vi "closeConfigFile.vi"(8 "error in (no error)":errorcluster, 11 "Path in":T1) -> (0 "error out":errorcluster)   [LabVIEW 2018]
doc: "Close the default.ini file.\n\nNOTE: this is only for internal use. User does not call this function directly."
uses:
  <vilib>/Utility/config.llb/Config Data RefNum.ctl
  <vilib>/Utility/config.llb/NI_LVConfig.lvlib
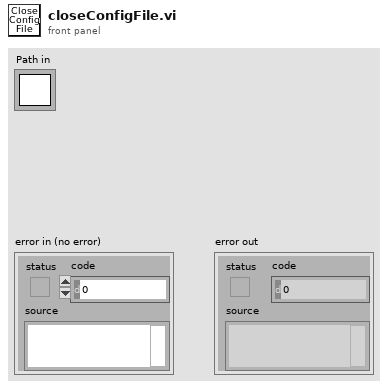
[diagram p1: front panel]
types:
  T1 = typedef "NI_LVConfig.lvlib/Config Data RefNum.ctl" = refnum<k1>
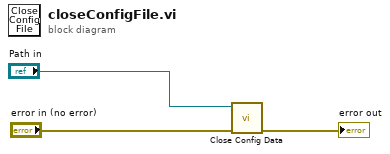
[diagram p0: block diagram]
diagram:
  n1 = call <vilib>:"Close Config Data.vi"("error in (no error)"="error in (no error)", "refnum"="Path in") -> ("error out"=→"error out":errorcluster)  [unwired: 8 in, 1 out]
